vi "VG_DCIRmax_P.vi"() -> ()   [LabVIEW 2020]
panel:
  out "DCIRmax":dbl
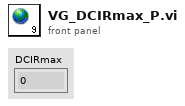
[diagram p1: front panel]
diagram:
